vi "Read Digital Waveform.vi"(8 "error in (no error)":errorcluster {"code" format="%.0x"}, 10 "Channel Name (\"POD1\")":string(combo)="POD1", 11 "VISA Resource Name":refnum<visa-resource-name>) -> (0 "error out":errorcluster {"code" format="%.0x"}, 1 "x increment":dbl caption="x Increment" format="%^.2e", 2 "initial x":dbl caption="Initial x" format="%^.2e", 3 "VISA Resource Name Out":refnum<visa-resource-name>, 4 "waveform array":u16[](array[numeric]) caption="Waveform Array", 5 "actual points":u32 caption="Actual Points")   [LabVIEW 2011, in "Agilent 546XX Series.lvlib"]
doc: "This VI initiates an acquisition on the digital channels that you enable with the ag546xx Configure Digital Channel VI. It then waits for the acquisition to complete, and returns the waveform for the digital channel you specify. You call the ag546xx Fetch Digital Waveform Single VI or ag546xx Fetch Digital Waveform Both VI to obtain the waveforms for each of the remaining enabled digital channels without initiating another acquisition.\n\nNotes:\n\n(1) This VI returns the digital waveforms in PODs of digital channels 0 to 7, 8 to 15, or 0 to 15.\n\n(2) If a single POD is chosen as the source, then the Waveform Array is returned as an unsigned 8 bit number with digital channels 7 or 15 as the most significant bit and digital channels 0 or 8 as the least significant bit, respectively. \n\n(3) If both PODs are chosen as the source, then the Waveform Array is returned as an unsigned 16 bit number with digital channel 15 as the most significant bit and digital channel 0 as the least significant bit.\n\n(4) This VI is only used by models 546xx\"D\" models."
uses:
  Agilent 546XX Series.lvlib
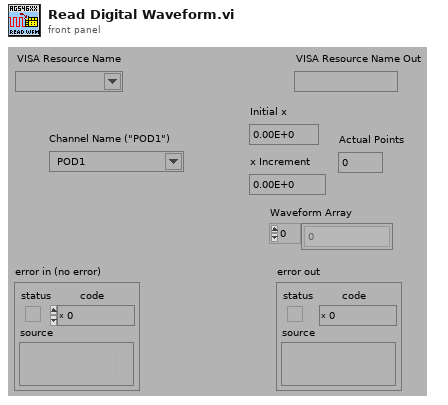
[diagram p1: front panel]
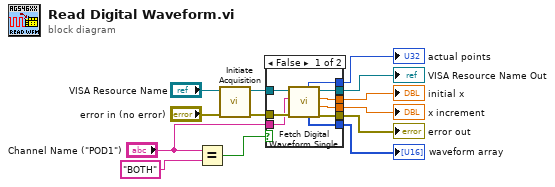
[diagram p0: block diagram]
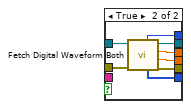
[diagram p2: hidden frame]
diagram:
  n1 = Equal?(x="Channel Name (\"POD1\")", y="BOTH" ("x")) -> (x = y?=w13:bool)
  n2 = call "Initiate Acquisition.vi"("error in (no error)"="error in (no error)", "VISA Resource Name"="VISA Resource Name") -> ("error out"=w9:errorcluster, "VISA Resource Name Out"=w12:refnum<visa-resource-name>)  [unwired: 8 in]
  n3 = case shown="False" w13 {
    tunnel: w12 -> [w21 w30]
    tunnel: w9 -> [w22 w29]
    tunnel: [w19 w28] -> w4
    tunnel: [w18 w27] -> w3
    tunnel: "Channel Name (\"POD1\")" -> [w20 _]
    tunnel: [w17 w26] -> w6
    tunnel: [w16 w25] -> w5
    tunnel: [w15 w24] -> w2
    tunnel: [w14 w23] -> w1
    frame False {
      n4 = call "Fetch Digital Waveform Single.vi"("error in (no error)"=w22, "Channel Name (\"POD1\")"=w20, "VISA Resource Name"=w21) -> ("error out"=w18:errorcluster, "x increment"=w16:dbl, "initial x"=w17:dbl, "VISA Resource Name Out"=w19:refnum<visa-resource-name>, "waveform array"=w15:u16[], "actual points"=w14:u32)  [unwired: 3 in]
    }
    frame True {
      n5 = call "Fetch Digital Waveform Both.vi"("error in (no error)"=w29, "VISA Resource Name"=w30) -> ("error out"=w27:errorcluster, "x increment"=w25:dbl, "initial x"=w26:dbl, "VISA Resource Name Out"=w28:refnum<visa-resource-name>, "waveform array"=w24:u16[], "actual points"=w23:u32)  [unwired: 4 in]
    }
  }
  "error out" <- w3
  "VISA Resource Name Out" <- w4
  "actual points" <- w1
  "initial x" <- w6
  "x increment" <- w5
  "waveform array" <- w2
